vi "OneSessTwoPinOneInstrOneSiteReservation_CallGetConnectionsFromPinsForTwoPinsAllSites_ReturnsTwoConnections.vi"() -> (0 "error out":errorcluster, 2 "result":string, 3 "pass":bool)   [LabVIEW 2020, in "MeasurementServerTests.lvlib"]
uses:
  MeasurementServerTests.lvlib
  Runtime/MeasurementLink Session Management/Session Reservation/Connection.ctl
  Runtime/MeasurementLink Session Management/Session Reservation/Hardware Independent Connection.ctl
  c3cb69a0-23cd-49fc-99d1-8c54773f0200.vi
  b3e5c3be-b7a7-4b6e-86ee-709eea9cb752.vi
  Runtime/MeasurementLink Session Management/Session Reservation/Get Connections Impl.vi
  Runtime/MeasurementLink Session Management/Session Reservation/Session Reservation.lvclass
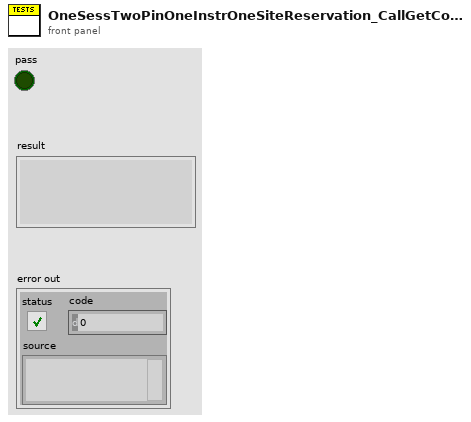
[diagram p1: front panel]
types:
  T1 = typedef "MeasurementLink Session Management.lvlib/Session Reservation.lvclass/Connection.ctl" = cluster{"connection":T2, "session":variant}
  T2 = typedef "MeasurementLink Session Management.lvlib/Session Reservation.lvclass/Hardware Independent Connection.ctl" = cluster{"pin or relay name":string, "site":i32, "instrument type id":string, "channel":string}
  T3 = typedef "MeasurementLink Session Management.lvlib/Session Reservation.lvclass/Data.ctl" = cluster{"session and driver infos":T4[], "pins":string[]}
  T4 = typedef "MeasurementLink Session Management.lvlib/Session Reservation.lvclass/Session and Driver Info.ctl" = cluster{"session info":T5, "session created":bool, "session":variant}
  T5 = typedef "MeasurementLink Session Management Client.lvlib/ni_measurementlink_sessionmanagement_v1_SessionInformation.ctl" = cluster{"session":T6, "resource_name":string, "channel_list":string, "instrument_type_id":string, "session_exists":bool, "channel_mappings":T7[]}
  T6 = typedef "MeasurementLink Session Management Client.lvlib/nidevice_grpc_Session.ctl" = cluster{"name":string}
  T7 = typedef "MeasurementLink Session Management Client.lvlib/ni_measurementlink_sessionmanagement_v1_ChannelMapping.ctl" = cluster{"pin_or_relay_name":string, "site":i32, "channel":string}
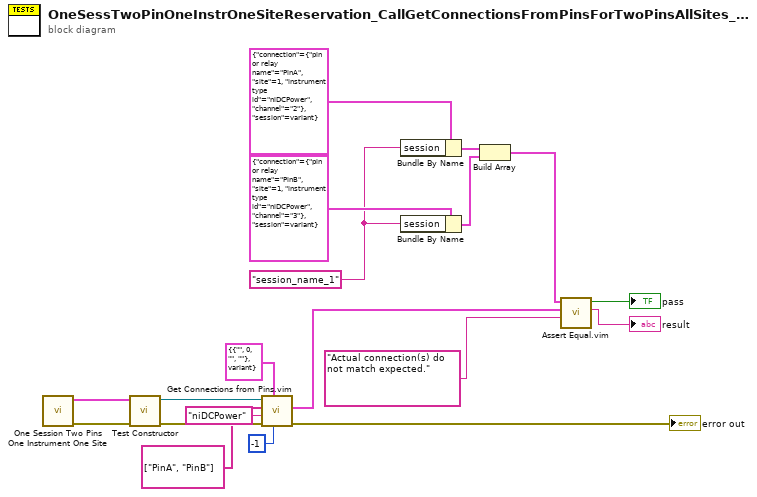
[diagram p0: block diagram]
diagram:
  w5 = "session_name_1"
  n1 = call "One Session Two Pins One Instrument One Site.vi"() -> ("error out"=w9:errorcluster, "data out"=w8:T3)  [unwired: 10 in]
  n2 = call "Test Constructor.vi"("error in"=w9, "data"=w8) -> ("error out"=w18:errorcluster, "Session Reservation out"=w17:refnum<class "Session Reservation.lvclass">)  [unwired: 8 in]
  n3 = call "Get Connections from Pins.vim"("site"=-1, "connection type"=T1 {"connection"={"pin or relay name"="", "site"=0, "instrument type id"="", "channel"=""}, "session"=variant} ("connection"), "error in"=w18, "instrument type id"="niDCPower", "pin or relay names"=string[] ["PinA", "PinB"], "session reservation in"=w17) -> ("error out"=→"error out":errorcluster, "connections"=w14:T1[])  [unwired: 3 in, 1 out]
  n4 = Bundle By Name(cluster=T1 {"connection"={"pin or relay name"="PinA", "site"=1, "instrument type id"="niDCPower", "channel"="2"}, "session"=variant} ("connection type"), "session"=w5) -> (w4:T1)
  n5 = Bundle By Name(cluster=T1 {"connection"={"pin or relay name"="PinB", "site"=1, "instrument type id"="niDCPower", "channel"="3"}, "session"=variant} ("connection type"), "session"=w5) -> (w3:T1)
  n6 = Build Array(w4, w3) -> (w2:T1[])
  n7 = call "Assert Equal.vim"("failure message"="Actual connection(s) do not match expected.", "actual value"=w14, "expected value"=w2) -> ("message"=→"result":string, "equal?"=→"pass":bool)  [unwired: 7 in]
